vi "Status_SendAsync.vi"(9 "Message":string, 11 "Database RefNum in":T1) -> ()   [LabVIEW 2016]
uses:
  DBSHAND/private/vis/DatabaseHand_RefNum.ctl
  DBSHAND/private/vis/DatabaseHand_Element_Get(string).vi
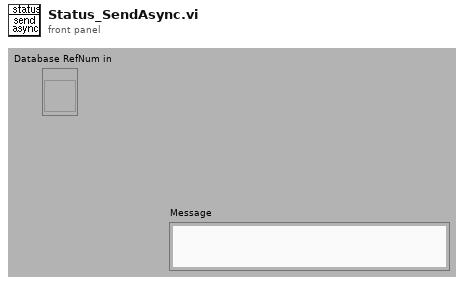
[diagram p1: front panel]
types:
  T1 = typedef "DatabaseHand_RefNum.ctl" = refnum<vi>
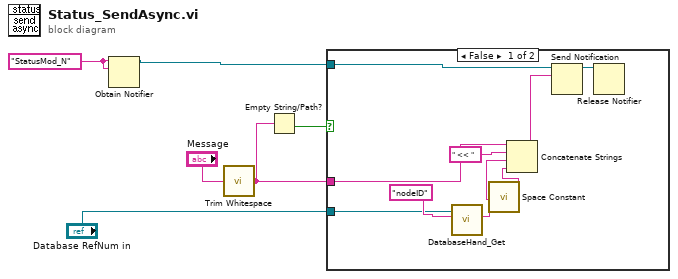
[diagram p0: block diagram]
diagram:
  w3 = "StatusMod_N" ("name (unnamed)")
  n1 = Obtain Notifier(name (unnamed)=w3, notification data type=w3) -> (notifier out=w2:refnum<notifier>)  [unwired: 2 in, 2 out]
  n2 = call <vilib>:"Trim Whitespace.vi"("string"="Message") -> ("trimmed string"=w5:string)  [unwired: 1 in]
  n3 = Empty String/Path?(string/path=w5) -> (empty?=w4:bool)
  n4 = case shown="False" w4 {
    tunnel: w5 -> [w13 _]
    tunnel: w2 -> [w12 _]
    tunnel: "Database RefNum in" -> [w7 _]
    frame False {
      n5 = call-poly "DatabaseHand_Get.vi"("name"="nodeID", "Database RefNum in"=w7) -> ("value"=w9:string)  [unwired: 3 in, 6 out]
      n6 = call <vilib>:"Space Constant.vi"() -> ("String"=w8:string)
      n7 = Concatenate Strings(w13, " << " ("string"), w9, w8) -> (w15:string)
      n8 = Send Notification(notification=w15, notifier=w12) -> (notifier out=w14:refnum<notifier>)  [unwired: 1 in, 1 out]
      n9 = Release Notifier(notifier=w14) -> ()  [unwired: 1 in, 4 out]
    }
    frame True {
    }
  }
